vi "BallShooter_Begin.vi"(8 "error in (no error)":errorcluster) -> (0 "error out":errorcluster)   [LabVIEW 2020]
doc: "Perform initialization actions for the ball shooter system."
uses:
  <vilib>/Rock Robotics/SystemInterfaces/DIO/FPGA_DIOChannel.ctl
  <vilib>/Rock Robotics/WPI/Relay/WPI_RelayDirection.ctl
  <vilib>/Rock Robotics/SystemInterfaces/DIO/FPGA_DIORelayChannel.ctl
  <vilib>/Rock Robotics/WPI/Switch/WPI_SwitchOpenLimit.vi
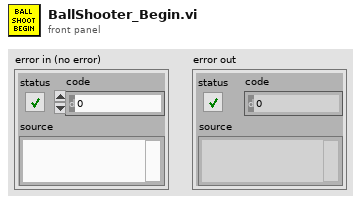
[diagram p1: front panel]
types:
  T1 = typedef "FPGA_DIOChannel.ctl" = enum8{"DIO 0", "DIO 1", "DIO 2", "DIO 3", "DIO 4", "DIO 5", "DIO 6", "DIO 7", "DIO 8", "DIO 9", "DIO MXP 0", "DIO MXP 1", "DIO MXP 2", "DIO MXP 3", "DIO MXP 4", "DIO MXP 5", "DIO MXP 6", "DIO MXP 7", "DIO MXP 8", "DIO MXP 9", "DIO MXP 10", "DIO MXP 11", "DIO MXP 12", "DIO MXP 13", "DIO MXP 14", "DIO MXP 15", "SPI Port CS1", "SPI Port CS2", "SPI Port CS3", "SPI Port MISO", "SPI Port MOSI", "Invalid"}
  T2 = typedef "WPI_RelayDirection.ctl" = enum16{"Both directions", "Forward only", "Reverse only"}
  T3 = typedef "FPGA_DIORelayChannel.ctl" = enum8{"Relay 0", "Relay 1", "Relay 2", "Relay 3", "Invalid"}
  T4 = typedef "WPI_SwitchDevRef.ctl" = cluster{"DevStatus":errorcluster, "DIO Channel":T1, "CntIndex":T5, "Normally Closed":bool}
  T5 = typedef "FPGA_CounterCtrSystemIndex.ctl" = enum8{"Ctr 0", "Ctr 1", "Ctr 2", "Ctr 3", "Ctr 4", "Ctr 5", "Ctr 6", "Ctr 7", "Invalid"}
  T6 = typedef "WPI_DigitalOutputDevRef.ctl" = cluster{"DIO Channel":T1, "DevStatus":errorcluster}
  T7 = typedef "WPI_RelayDevRef.ctl" = cluster{"DevStatus":errorcluster, "Relay Channel":T3, "Relay Direction":T2}
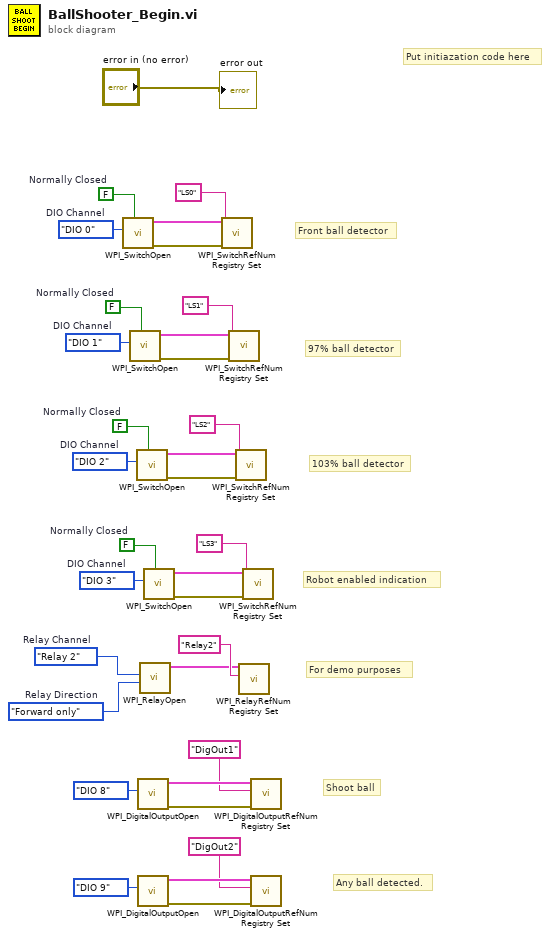
[diagram p0: block diagram]
diagram:
  w33 = WPI_RelayDirection."Forward only"  # Relay Direction
  w32 = FPGA_DIORelayChannel."Relay 2"  # Relay Channel
  w26 = FALSE  # Normally Closed
  w25 = FPGA_DIOChannel."DIO 3"  # DIO Channel
  w21 = FALSE  # Normally Closed
  w20 = FPGA_DIOChannel."DIO 2"  # DIO Channel
  w16 = FALSE  # Normally Closed
  w15 = FPGA_DIOChannel."DIO 1"  # DIO Channel
  w11 = FALSE  # Normally Closed
  w10 = FPGA_DIOChannel."DIO 0"  # DIO Channel
  # "Any ball detected."
  # "Shoot ball"
  # "For demo purposes"
  # "Robot enabled indication"
  # "103% ball detector"
  # "97% ball detector"
  # "Front ball detector"
  # "Put initiazation code here"
  n1 = call-poly <vilib>:"WPI_SwitchOpen.vi"("Normally Closed"=w11, "DIO Channel"=w10) -> ("error out"=w13:errorcluster, "SwitchDevRef"=w12:T4)  [unwired: 8 in]
  n2 = call-poly <vilib>:"WPI_SwitchOpen.vi"("Normally Closed"=w16, "DIO Channel"=w15) -> ("error out"=w18:errorcluster, "SwitchDevRef"=w17:T4)  [unwired: 8 in]
  n3 = call-poly <vilib>:"WPI_SwitchOpen.vi"("Normally Closed"=w21, "DIO Channel"=w20) -> ("error out"=w23:errorcluster, "SwitchDevRef"=w22:T4)  [unwired: 8 in]
  n4 = call <vilib>:"WPI_DigitalOutputOpen.vi"("DIO Channel"=FPGA_DIOChannel."DIO 8") -> ("error out"=w6:errorcluster, "DigitalOutputDevRef"=w7:T6)  [unwired: 9 in]
  n5 = call <vilib>:"WPI_DigitalOutputOpen.vi"("DIO Channel"=FPGA_DIOChannel."DIO 9") -> ("error out"=w2:errorcluster, "DigitalOutputDevRef"=w3:T6)  [unwired: 9 in]
  n6 = call <vilib>:"WPI_RelayOpen.vi"("Relay Direction"=w33, "Relay Channel"=w32) -> ("RelayDevRef"=w30:T7)  [unwired: 8 in, 1 out]
  n7 = call-poly <vilib>:"WPI_SwitchOpen.vi"("Normally Closed"=w26, "DIO Channel"=w25) -> ("error out"=w28:errorcluster, "SwitchDevRef"=w27:T4)  [unwired: 8 in]
  n8 = call <vilib>:"WPI_SwitchRefNum Registry Set.vi"("error in (no error)"=w13, "refnum name"="LS0", "SwitchDevRef"=w12) -> ()  [unwired: 7 in, 2 out]
  n9 = call <vilib>:"WPI_SwitchRefNum Registry Set.vi"("error in (no error)"=w18, "refnum name"="LS1", "SwitchDevRef"=w17) -> ()  [unwired: 7 in, 2 out]
  n10 = call <vilib>:"WPI_SwitchRefNum Registry Set.vi"("error in (no error)"=w23, "refnum name"="LS2", "SwitchDevRef"=w22) -> ()  [unwired: 7 in, 2 out]
  n11 = call <vilib>:"WPI_RelayRefNum Registry Set.vi"("refnum name"="Relay2", "RelayDevRef"=w30) -> ()  [unwired: 8 in, 2 out]
  n12 = call <vilib>:"WPI_SwitchRefNum Registry Set.vi"("error in (no error)"=w28, "refnum name"="LS3", "SwitchDevRef"=w27) -> ()  [unwired: 7 in, 2 out]
  n13 = call <vilib>:"WPI_DigitalOutputRefNum Registry Set.vi"("error in (no error)"=w6, "refnum name"="DigOut1", "DigitalOutputDevRef"=w7) -> ()  [unwired: 7 in, 2 out]
  n14 = call <vilib>:"WPI_DigitalOutputRefNum Registry Set.vi"("error in (no error)"=w2, "refnum name"="DigOut2", "DigitalOutputDevRef"=w3) -> ()  [unwired: 7 in, 2 out]
  "error out" <- "error in (no error)"
